vi "LabVIEW_MQTT_Toolkit_V2.vi"() -> ()   [LabVIEW 2021] (continued)
            n1097 = Array Subset(array=w2829, index=2, length=8) -> (w2869:u8[])
            n1098 = Subtract(x=w2830, y=36) -> (x-y=w2825:i32)
            n1099 = Unbundle By Name(w2864) -> ("[0]"=w2863:u8)
            n1100 = Array To Cluster(array=w2869) -> (cluster=w2868:T12)
            n1101 = Unbundle By Name(w2859) -> ("[0]"=w2858:u8, "[1]"=w2729:u8, "[2]"=w2857:u8, "[3]"=w2854:u8, "[4]"=w2853:u8, "[5]"=w2851:u8, "[6]"=w2850:u8, "[7]"=w2849:u8, "[8]"=w2846:u8, "[9]"=w2845:u8, "[10]"=w2844:u8, "[11]"=w2841:u8, "[12]"=w2840:u8, "[13]"=w2834:u8, "[14]"=→"Network quality (LQI)":u8, "[15]"=w2726:u8, "[16]"=w2712:u8, "[17]"=w2711:u8, "[18]"=w2710:u8, "[19]"=w2709:u8, "[20]"=w2702:u8, "[21]"=w2701:u8)
            n1102 = Array Subset(array=w2829, index=36, length=w2825) -> (w2827:u8[])
            n1103 = Unbundle By Name(w2868) -> ("[0]"=w2810:u8, "[1]"=w2811:u8, "[2]"=w2814:u8, "[3]"=w2815:u8, "[4]"=w2808:u8, "[5]"=w2809:u8, "[6]"=w2817:u8, "[7]"=w2816:u8)
            n1104 = case shown="Default" w2726 {
              tunnel: ["channel Z" "channel X" _ "channel Y"] -> w2725
              frame 0 {
              }
              frame 1 {
              }
              frame Default {
              }
              frame 2 {
              }
            }
            "Shock source" <- w2725
            n1105 = Join Numbers "time"(hi=w2811, lo=w2810) -> ((hi.lo)=w2807:u16)
            n1106 = Join Numbers "date"(hi=w2815, lo=w2814) -> ((hi.lo)=w2813:u16)
            n1107 = Join Numbers(hi=w2850, lo=w2851) -> ((hi.lo)=w2848:u16)
            n1108 = Join Numbers(hi=w2845, lo=w2846) -> ((hi.lo)=w2843:u16)
            n1109 = Join Numbers(hi=w2816, lo=w2817) -> ((hi.lo)=w2818:u16)
            n1110 = Join Numbers(hi=w2853, lo=w2854) -> ((hi.lo)=w2852:u16)
            n1111 = Join Numbers(hi=w2729, lo=w2858) -> ((hi.lo)=w2856:u16)
            n1112 = Join Numbers(hi=w2840, lo=w2841) -> ((hi.lo)=w2839:u16)
            n1113 = Join Numbers(hi=w2711, lo=w2712) -> ((hi.lo)=w2720:u16)
            n1114 = Join Numbers(hi=w2709, lo=w2710) -> ((hi.lo)=w2714:u16)
            n1115 = Join Numbers(hi=w2701, lo=w2702) -> ((hi.lo)=w2704:u16)
            n1116 = Join Numbers(hi=w2809, lo=w2808) -> ((hi.lo)=w2800:u16)
            "millisec" <- w2800
            n1117 = Not Equal To 0?(x=w2834) -> (x != 0?=→"synchronised":bool)
            n1118 = Equal To 0?(x=w2834) -> (x = 0?=→"not synchronised":bool)
            n1119 = Decimate 1D Array(w2827) -> (w2820:u8[], w2826:u8[], w2824:u8[])
            n1120 = Join Numbers(hi=w2849, lo=w2848) -> ((hi.lo)=w2847:u32)
            n1121 = Join Numbers(hi=w2844, lo=w2843) -> ((hi.lo)=w2842:u32)
            n1122 = Join Numbers(hi=w2826, lo=w2820) -> ((hi.lo)=w2823:u16[])
            n1123 = Join Numbers(hi=w2857, lo=w2856) -> ((hi.lo)=w2855:u32)
            n1124 = To Word Integer(number=w2839) -> (16bit integer=→"Prev.number of daq per channel":i16)
            n1125 = To Word Integer(number=w2720) -> (16bit integer=w2719:i16)
            n1126 = To Word Integer(number=w2714) -> (16bit integer=w2713:i16)
            n1127 = To Word Integer(number=w2704) -> (16bit integer=w2703:i16)
            n1128 = To Word Integer(number=w2852) -> (16bit integer=w2821:i16)
            "Number of daq per channel" <- w2821
            n1129 = And(x=w2713, y=w2715) -> (x .and. y?=w2716:i16)
            n1130 = And(x=w2703, y=w2705) -> (x .and. y?=w2706:i16)
            n1131 = And(x=w2719, y=w2721) -> (x .and. y?=w2722:i16)
            n1132 = To Long Integer(number=w2847) -> (32bit integer=w2751:i32)
            "Data monitoring cycle" <- w2751
            n1133 = To Long Integer(number=w2842) -> (32bit integer=w2752:i32)
            "Data acquisition duration" <- w2752
            n1134 = To Long Integer(number=w2855) -> (32bit integer=w2822:i32)
            "Frame sequence Id" <- w2822
            n1135 = Divide(x=w2800, y=i16 1000) -> (x/y=w2801:dbl)
            n1136 = for {
              tunnel: w2824 -> [w3352] mode=indexing
              tunnel: [w3350] -> w2780 mode=indexing
              tunnel: w2823 -> [w3348] mode=indexing
              n1137 = To Word Integer(number=w3352) -> (16bit integer=w3349:i16)
              n1138 = Sign(1:w3349) -> (0:w3351:i16)
              n1139 = case shown="1" w3351 {
                tunnel: [_ w3354 w3357] -> w3350
                tunnel: w3348 -> [_ w3353 w3356]
                frame Default {
                }
                frame 1 {
                  n1140 = Divide(x=w3353, y=-1000.0) -> (x/y=w3354:dbl)
                }
                frame 0 {
                  n1141 = Divide(x=w3356, y=1000.0) -> (x/y=w3357:dbl)
                }
              }
            }
            n1142 = And(x=i16 -32768 ("Numeric"), y=w2722) -> (x .and. y?=w2723:i16)
            n1143 = To Unsigned Word Integer(number=w2801) -> (unsigned 16bit integer=w2805:u16)
            n1144 = case shown="4" w2837 {
              tunnel: ["" "LDCDA mode" "Shock Detection"] -> w2775
              tunnel: w2752 -> [_ _ _]
              tunnel: w2751 -> [_ _ _]
              frame Default {
              }
              frame 1 {
              }
              frame 4 {
              }
            }
            n1145 = case shown="0" w2723 {
              tunnel: [w2889 w2890] -> w2699
              tunnel: w2722 -> [w2889 w2895]
              tunnel: w2721 -> [_ w2891]
              frame 0 {
                # "positive"
              }
              frame Default {
                # "negative"
                n1146 = Not(x=w2895) -> (.not. x?=w2894:i16)
                n1147 = And(x=w2894, y=w2891) -> (x .and. y?=w2892:i16)
                n1148 = Increment(x=w2892) -> (x+1=w2893:i16)
                n1149 = Negate(x=w2893) -> (-x=w2890:i16)
              }
            }
            n1150 = Multiply(x=w2821, y=w2822) -> (x*y=w2794:i32)
            n1151 = And(x=i16 -32768 ("Numeric"), y=w2716) -> (x .and. y?=w2717:i16)
            n1152 = And(x=i16 -32768 ("Numeric"), y=w2706) -> (x .and. y?=w2707:i16)
            n1153 = Add(x=w2807, y=w2805) -> (x+y=w2779:u16)
            n1154 = To Unsigned Word Integer(number=w2813) -> (unsigned 16bit integer=w2778:u16)
            n1155 = case shown="0" w2717 {
              tunnel: [w2882 w2883] -> w2695
              tunnel: w2716 -> [w2882 w2888]
              tunnel: w2715 -> [_ w2884]
              frame 0 {
                # "positive"
              }
              frame Default {
                # "negative"
                n1156 = Not(x=w2888) -> (.not. x?=w2887:i16)
                n1157 = And(x=w2887, y=w2884) -> (x .and. y?=w2885:i16)
                n1158 = Increment(x=w2885) -> (x+1=w2886:i16)
                n1159 = Negate(x=w2886) -> (-x=w2883:i16)
              }
            }
            n1160 = case shown="0" w2707 {
              tunnel: [w2875 w2876] -> w2692
              tunnel: w2706 -> [w2875 w2881]
              tunnel: w2705 -> [_ w2877]
              frame 0 {
                # "positive"
              }
              frame Default {
                # "negative"
                n1161 = Not(x=w2881) -> (.not. x?=w2880:i16)
                n1162 = And(x=w2880, y=w2877) -> (x .and. y?=w2878:i16)
                n1163 = Increment(x=w2878) -> (x+1=w2879:i16)
                n1164 = Negate(x=w2879) -> (-x=w2876:i16)
              }
            }
            n1165 = Join Numbers(hi=w2778, lo=w2779) -> ((hi.lo)=w2812:u32)
            n1166 = To Unsigned Byte Integer(number=w2863) -> (unsigned 8bit integer=w2782:u8)
            n1167 = To Unsigned Quad Integer(1:w2794) -> (0:w2793:u64)
            n1168 = case shown="6" w2796 {
              tunnel: ["AX-3D" "HI_INC_MONO" "HI_INC_BI" "X_INC_MONO " "X _INC_BI " "AX_3DS" ""] -> w2727
              frame 1 {
              }
              frame 2 {
              }
              frame 3 {
              }
              frame 4 {
              }
              frame 5 {
              }
              frame 6 {
              }
              frame Default {
              }
            }
            "Device type" <- w2727
            n1169 = To Unsigned Quad Integer(1:w2812) -> (0:w2806:u64)
            n1170 = Increment(x=w2793) -> (x+1=w2797:u64)
            n1171 = for {
              N: w2797 -> [_]
              tunnel: w2793 -> [w3347]
              tunnel: [w3347] -> w2799
            }
            n1172 = call "Unix Time to Timestamp.vi"("Fractional Second"=w2801, "Unix Time (s)"=w2806) -> ("Timestamp"=w2803:timestamp)  [unwired: 8 in, 1 out]
            n1173 = To Word Integer(number=w2818) -> (16bit integer=w2753:i16)
            "Sampling rate" <- w2753
            n1174 = Format Date/Time String(time format string (%c)="%x %X %3u", seconds (now)=w2803, UTC format=TRUE) -> (date/time string=w2745:string)
            "Ref time" <- w2745
            n1175 = Decrement(x=w2799) -> (x-1=w2798:u64)
            n1176 = call <vilib>:"Space Constant.vi"() -> ("String"=w2700:string)
            n1177 = Search and Replace String(replace all?=TRUE ("replace all? (F)"), input string=w2745, search string=":", replace string="_") -> (result string=w2766:string)  [unwired: 4 in, 3 out]
            n1178 = Divide(x=w2699, y=i16 1000) -> (x/y=→"Y Axis first data":dbl)
            n1179 = Number To Decimal String(number=w2753) -> (decimal integer string=w2742:string)  [unwired: 1 in]
            n1180 = Number To Decimal String(number=w2751) -> (decimal integer string=w2739:string)  [unwired: 1 in]
            n1181 = Number To Decimal String(number=w2752) -> (decimal integer string=w2736:string)  [unwired: 1 in]
            n1182 = Concatenate Strings(w2775, w2700) -> (w2728:string)
            "Measure mode" <- w2728
            n1183 = for {
              tunnel: w2780 -> [w3346] mode=indexing
              shift-right: [w3344] -> _
              shift-left: w2798 -> [w3345]
              tunnel: [w3343] -> w2795 mode=indexing
              tunnel: [w3346] -> _ mode=indexing
              n1184 = Increment(x=w3345) -> (x+1=w3344:u64)
              n1185 = To Unsigned Quad Integer(1:w3344) -> (0:w3343:u64)
            }
            n1186 = Search and Replace String(replace all?=TRUE ("replace all? (F)"), input string=w2766, search string=",", replace string="_") -> (result string=w2765:string)  [unwired: 4 in, 3 out]
            n1187 = Divide(x=w2695, y=i16 1000) -> (x/y=→"X Axis first data":dbl)
            n1188 = Divide(x=w2692, y=i16 1000) -> (x/y=→"Z Axis first data":dbl)
            n1189 = Concatenate Strings("Device type :", w2727, ";", "Measure Mode :", w2728, ";", "Reference time :" ("string"), w2745, ";", " Sampling rate :", w2742, ";" ("string"), "Data monitoring cycle" ("string"), w2739, ";" ("string"), "Data acquisition duration :" ("string"), w2736, ";" ("string"), "\n") -> (w2755:string)
            n1190 = Search and Replace String(replace all?=TRUE ("replace all? (F)"), input string=w2765, search string="/", replace string="_") -> (result string=w2761:string)  [unwired: 4 in, 3 out]
            n1191 = String Subset(string=w2761, offset (0)=0, length (rest)=20 ("length (rest)")) -> (substring=w2758:string)
            n1192 = To Double Precision Float(number=w2753) -> (double precision float=w2776:dbl)
            n1193 = Build Array(w2755) -> (w2750:string[])
            n1194 = call <vilib>:"Space Constant.vi"() -> ("String"=w2757:string)
            n1195 = Concatenate Strings(w2758, "_" ("string"), w2730, w2757) -> (w2771:string)
            n1196 = To Unsigned Quad Integer(1:w2795) -> (0:w2777:u64[])
            n1197 = case shown="101" w2782 {
              tunnel: ["" "no active channel" "chZ " "chX  " "chZ & chX " "chY" "chZ & chY  " "chX & chY " "chZ& chX& chY "] -> w2781
              tunnel: w2780 -> [_ _ w2935 w2994 w3055 w3117 w3179 w3244 w3312]
              tunnel: [_ _ w2932 w2991 w3051 w3114 w3177 w3240 w3308] -> w2754
              tunnel: w2777 -> [_ _ w2934 w2993 w3054 w3115 w3178 w3243 w3307]
              tunnel: [_ _ w2931 _ w3050 _ w3174 _ w3306] -> w2788
              tunnel: [_ _ _ w2990 w3049 _ _ w3239 w3305] -> w2787
              tunnel: [_ _ _ _ _ w3113 w3173 w3238 w3304] -> w2786
              tunnel: w2779 -> [_ _ w2930 w2988 w3047 w3111 w3171 w3236 w3302]
              tunnel: w2778 -> [_ _ w2929 w2989 w3048 w3112 w3172 w3237 w3303]
              tunnel: w2777 -> [_ _ w2928 w2987 w3046 w3110 w3170 w3235 w3301]
              tunnel: w2776 -> [_ _ w2927 w2986 w3045 w3109 w3169 w3234 w3300]
              tunnel: [_ _ w2926 _ w3044 _ w3168 _ w3299] -> w2785
              tunnel: [_ _ _ w2985 w3044 _ _ w3233 w3298] -> w2784
              tunnel: [_ _ _ _ _ w3108 w3167 w3232 w3297] -> w2783
              tunnel: w2771 -> [_ _ w2912 w2962 w3021 w3085 w3143 w3209 w3274]
              tunnel: [_ _ w2902 w2961 w3020 w3084 w3144 w3208 w3273] -> w2689
              tunnel: w2750 -> [_ _ w2901 w2960 w3019 w3083 w3142 w3207 w3272]
              frame Default {
              }
              frame 0 {
              }
              frame 1 {
                w2907 = T14 2 items=["User Home"=0, "User Desktop"=1, "User Documents"=2, "User Application Data"=3, "User Preferences"=4, "User Temporary"=5, "Public Documents"=6, "Public Application Data"=7, "Public Preferences"=8, "Public Cache"=13, "System Core Libraries"=9, "System Installed Libraries"=10, "Application Files"=11, "Boot Volume Root"=12] ("system directory type")
                n1198 = Decimate 1D Array(w2935) -> (w2933:dbl[])
                n1199 = Search and Replace String(replace all?=TRUE ("replace all? (F)"), input string=w2912, search string="/") -> (result string=w2924:string)  [unwired: 5 in, 3 out]
                n1200 = Concatenate Strings(w2901, "TimeStamp;MeasureCh_Z(g);", "\n") -> (w2917:string)
                n1201 = for {
                  tunnel: w2933 -> [w2954] mode=indexing
                  tunnel: [w2957] -> w2932 mode=indexing
                  tunnel: w2934 -> [w2956] mode=indexing
                  tunnel: [w2954] -> w2931 mode=indexing
                  tunnel: w2930 -> [w2949]
                  tunnel: w2929 -> [w2948]
                  tunnel: w2928 -> [w2947] mode=indexing
                  tunnel: w2927 -> [w2946]
                  tunnel: [w2940] -> w2926
                  n1202 = Join Numbers(hi=w2948, lo=w2949) -> ((hi.lo)=w2951:u32)
                  n1203 = To Double Precision Float(number=w2947) -> (double precision float=w2952:dbl)
                  n1204 = Number To Decimal String(number=w2956) -> (decimal integer string=w2955:string)  [unwired: 1 in]
                  n1205 = Number To Fractional String(number=w2954, precision (6)=i16 3 ("width (-)")) -> (F-format string=w2958:string)  [unwired: 2 in]
                  n1206 = Divide(x=w2952, y=w2946) -> (x/y=w2953:dbl)
                  n1207 = Build Array(w2955, w2958) -> (w2957:string[])
                  n1208 = To Unsigned Quad Integer(1:w2951) -> (0:w2950:u64)
                  n1209 = call "Unix Time to Timestamp.vi"("Fractional Second"=w2953, "Unix Time (s)"=w2950) -> ("Timestamp"=w2941:timestamp)  [unwired: 8 in, 1 out]
                  n1210 = Format Date/Time String(seconds (now)=w2941, UTC format=TRUE) -> (date/time string=w2942:string)  [unwired: 1 in]
                  n1211 = Scan From String(format string="%<%x %H:%M:%S%3u>T", input string=w2942) -> (output 1=w2943:timestamp)  [unwired: 3 in, 3 out]
                  n1212 = To Double Precision Float(number=w2943) -> (double precision float=w2940:dbl)
                }
                n1213 = call <vilib>:"Get System Directory.vi"("system directory type"=w2907) -> ("system directory"=w2918:path)  [unwired: 10 in]
                n1214 = Concatenate Strings(w2924, "_" ("string"), "ShockDetection.csv") -> (w2925:string)
                n1215 = Build Path(base path=w2918, name or relative path="Logfile") -> (appended path=w2919:path)
                n1216 = call <vilib>:"Check if File or Folder Exists.vi"("path"=w2919) -> ("file or folder exists?"=w2920:bool, "dup path"=w2921:path)  [unwired: 8 in, 1 out]
                n1217 = case shown="False" w2920 {
                  tunnel: w2921 -> [w2938 w2939]
                  tunnel: [w2937 w2939] -> w2922
                  frame False {
                    n1218 = Create Folder(path (use dialog)=w2938) -> (created path=w2937:path)  [unwired: 2 in, 2 out]
                  }
                  frame True {
                  }
                }
                n1219 = Build Path(base path=w2922, name or relative path=w2925) -> (appended path=w2923:path)
                n1220 = Open/Create/Replace File(file path (use dialog)=w2923, operation (0:open)=T11."open or create") -> (refnum out=w2916:refnum<file>, error out=w2914:errorcluster)  [unwired: 4 in, 1 out]
                n1221 = Write to Text File(file (use dialog)=w2916, text=w2917, error in=w2914) -> (refnum out=w2915:refnum<file>, error out=w2913:errorcluster)  [unwired: 1 in, 1 out]
                n1222 = Close File(refnum=w2915, error in=w2913) -> (path=w2902:path)  [unwired: 1 out]
              }
              frame 2 {
                w2967 = T14 2 items=["User Home"=0, "User Desktop"=1, "User Documents"=2, "User Application Data"=3, "User Preferences"=4, "User Temporary"=5, "Public Documents"=6, "Public Application Data"=7, "Public Preferences"=8, "Public Cache"=13, "System Core Libraries"=9, "System Installed Libraries"=10, "Application Files"=11, "Boot Volume Root"=12] ("system directory type")
                n1223 = Decimate 1D Array(w2994) -> (w2992:dbl[])
                n1224 = Search and Replace String(replace all?=TRUE ("replace all? (F)"), input string=w2962, search string="/") -> (result string=w2983:string)  [unwired: 5 in, 3 out]
                n1225 = for {
                  tunnel: w2992 -> [w3013] mode=indexing
                  tunnel: [w3016] -> w2991 mode=indexing
                  tunnel: w2993 -> [w3015] mode=indexing
                  tunnel: [w3013] -> w2990 mode=indexing
                  tunnel: w2989 -> [w3008]
                  tunnel: w2988 -> [w3007]
                  tunnel: w2987 -> [w3006] mode=indexing
                  tunnel: w2986 -> [w3005]
                  tunnel: [w2999] -> w2985
                  n1226 = Join Numbers(hi=w3008, lo=w3007) -> ((hi.lo)=w3010:u32)
                  n1227 = To Double Precision Float(number=w3006) -> (double precision float=w3011:dbl)
                  n1228 = Number To Decimal String(number=w3015) -> (decimal integer string=w3014:string)  [unwired: 1 in]
                  n1229 = Number To Fractional String(number=w3013, precision (6)=i16 3 ("width (-)")) -> (F-format string=w3017:string)  [unwired: 2 in]
                  n1230 = Divide(x=w3011, y=w3005) -> (x/y=w3012:dbl)
                  n1231 = Build Array(w3014, w3017) -> (w3016:string[])
                  n1232 = To Unsigned Quad Integer(1:w3010) -> (0:w3009:u64)
                  n1233 = call "Unix Time to Timestamp.vi"("Fractional Second"=w3012, "Unix Time (s)"=w3009) -> ("Timestamp"=w3000:timestamp)  [unwired: 8 in, 1 out]
                  n1234 = Format Date/Time String(seconds (now)=w3000, UTC format=TRUE) -> (date/time string=w3001:string)  [unwired: 1 in]
                  n1235 = Scan From String(format string="%<%x %H:%M:%S%3u>T", input string=w3001) -> (output 1=w3002:timestamp)  [unwired: 3 in, 3 out]
                  n1236 = To Double Precision Float(number=w3002) -> (double precision float=w2999:dbl)
                }
                n1237 = Concatenate Strings(w2960, "TimeStamp;MeasureCh_X(g);", "\n") -> (w2976:string)
                n1238 = call <vilib>:"Get System Directory.vi"("system directory type"=w2967) -> ("system directory"=w2977:path)  [unwired: 10 in]
                n1239 = Concatenate Strings(w2983, "_" ("string"), "ShockDetection.csv") -> (w2984:string)
                n1240 = Build Path(base path=w2977, name or relative path="Logfile") -> (appended path=w2978:path)
                n1241 = call <vilib>:"Check if File or Folder Exists.vi"("path"=w2978) -> ("file or folder exists?"=w2979:bool, "dup path"=w2980:path)  [unwired: 8 in, 1 out]
                n1242 = case shown="False" w2979 {
                  tunnel: w2980 -> [w2997 w2998]
                  tunnel: [w2996 w2998] -> w2981
                  frame False {
                    n1243 = Create Folder(path (use dialog)=w2997) -> (created path=w2996:path)  [unwired: 2 in, 2 out]
                  }
                  frame True {
                  }
                }
                n1244 = Build Path(base path=w2981, name or relative path=w2984) -> (appended path=w2982:path)
                n1245 = Open/Create/Replace File(file path (use dialog)=w2982, operation (0:open)=T11."open or create") -> (refnum out=w2975:refnum<file>, error out=w2973:errorcluster)  [unwired: 4 in, 1 out]
                n1246 = Write to Text File(file (use dialog)=w2975, text=w2976, error in=w2973) -> (refnum out=w2974:refnum<file>, error out=w2972:errorcluster)  [unwired: 1 in, 1 out]
                n1247 = Close File(refnum=w2974, error in=w2972) -> (path=w2961:path)  [unwired: 1 out]
              }
              frame 3 {
                w3026 = T14 2 items=["User Home"=0, "User Desktop"=1, "User Documents"=2, "User Application Data"=3, "User Preferences"=4, "User Temporary"=5, "Public Documents"=6, "Public Application Data"=7, "Public Preferences"=8, "Public Cache"=13, "System Core Libraries"=9, "System Installed Libraries"=10, "Application Files"=11, "Boot Volume Root"=12] ("system directory type")
                n1248 = Decimate 1D Array(w3055) -> (w3053:dbl[], w3052:dbl[])
                n1249 = Search and Replace String(replace all?=TRUE ("replace all? (F)"), input string=w3021, search string="/") -> (result string=w3042:string)  [unwired: 5 in, 3 out]
                n1250 = for {
                  tunnel: w3053 -> [w3075] mode=indexing
                  tunnel: w3052 -> [w3074] mode=indexing
                  tunnel: [w3078] -> w3051 mode=indexing
                  tunnel: w3054 -> [w3077] mode=indexing
                  tunnel: [w3075] -> w3050 mode=indexing
                  tunnel: [w3074] -> w3049 mode=indexing
                  tunnel: w3048 -> [w3069]
                  tunnel: w3047 -> [w3068]
                  tunnel: w3046 -> [w3067] mode=indexing
                  tunnel: w3045 -> [w3066]
                  tunnel: [w3060] -> w3044
                  n1251 = Join Numbers(hi=w3069, lo=w3068) -> ((hi.lo)=w3071:u32)
                  n1252 = To Double Precision Float(number=w3067) -> (double precision float=w3072:dbl)
                  n1253 = Number To Decimal String(number=w3077) -> (decimal integer string=w3076:string)  [unwired: 1 in]
                  n1254 = Number To Fractional String(number=w3075, precision (6)=i16 3 ("width (-)")) -> (F-format string=w3080:string)  [unwired: 2 in]
                  n1255 = Number To Fractional String(number=w3074, precision (6)=i16 3 ("width (-)")) -> (F-format string=w3079:string)  [unwired: 2 in]
                  n1256 = Divide(x=w3072, y=w3066) -> (x/y=w3073:dbl)
                  n1257 = Build Array(w3076, w3080, w3079) -> (w3078:string[])
                  n1258 = To Unsigned Quad Integer(1:w3071) -> (0:w3070:u64)
                  n1259 = call "Unix Time to Timestamp.vi"("Fractional Second"=w3073, "Unix Time (s)"=w3070) -> ("Timestamp"=w3061:timestamp)  [unwired: 8 in, 1 out]
                  n1260 = Format Date/Time String(seconds (now)=w3061, UTC format=TRUE) -> (date/time string=w3062:string)  [unwired: 1 in]
                  n1261 = Scan From String(format string="%<%x %H:%M:%S%3u>T", input string=w3062) -> (output 1=w3063:timestamp)  [unwired: 3 in, 3 out]
                  n1262 = To Double Precision Float(number=w3063) -> (double precision float=w3060:dbl)
                }
                n1263 = Concatenate Strings(w3019, "TimeStamp;MeasureCh_Z(g);Ch_X(g);", "\n") -> (w3035:string)
                n1264 = call <vilib>:"Get System Directory.vi"("system directory type"=w3026) -> ("system directory"=w3036:path)  [unwired: 10 in]
                n1265 = Concatenate Strings(w3042, "_" ("string"), "ShockDetection.csv") -> (w3043:string)
                n1266 = Build Path(base path=w3036, name or relative path="Logfile") -> (appended path=w3037:path)
                n1267 = call <vilib>:"Check if File or Folder Exists.vi"("path"=w3037) -> ("file or folder exists?"=w3038:bool, "dup path"=w3039:path)  [unwired: 8 in, 1 out]
                n1268 = case shown="False" w3038 {
                  tunnel: w3039 -> [w3058 w3059]
                  tunnel: [w3057 w3059] -> w3040
                  frame False {
                    n1269 = Create Folder(path (use dialog)=w3058) -> (created path=w3057:path)  [unwired: 2 in, 2 out]
                  }
                  frame True {
                  }
                }
                n1270 = Build Path(base path=w3040, name or relative path=w3043) -> (appended path=w3041:path)
                n1271 = Open/Create/Replace File(file path (use dialog)=w3041, operation (0:open)=T11."open or create") -> (refnum out=w3034:refnum<file>, error out=w3032:errorcluster)  [unwired: 4 in, 1 out]
                n1272 = Write to Text File(file (use dialog)=w3034, text=w3035, error in=w3032) -> (refnum out=w3033:refnum<file>, error out=w3031:errorcluster)  [unwired: 1 in, 1 out]
                n1273 = Close File(refnum=w3033, error in=w3031) -> (path=w3020:path)  [unwired: 1 out]
              }
              frame 4 {
                w3090 = T14 2 items=["User Home"=0, "User Desktop"=1, "User Documents"=2, "User Application Data"=3, "User Preferences"=4, "User Temporary"=5, "Public Documents"=6, "Public Application Data"=7, "Public Preferences"=8, "Public Cache"=13, "System Core Libraries"=9, "System Installed Libraries"=10, "Application Files"=11, "Boot Volume Root"=12] ("system directory type")
                n1274 = Decimate 1D Array(w3117) -> (w3116:dbl[])
                n1275 = Search and Replace String(replace all?=TRUE ("replace all? (F)"), input string=w3085, search string="/") -> (result string=w3106:string)  [unwired: 5 in, 3 out]
                n1276 = for {
                  tunnel: w3116 -> [w3136] mode=indexing
                  tunnel: [w3139] -> w3114 mode=indexing
                  tunnel: w3115 -> [w3138] mode=indexing
                  tunnel: [w3136] -> w3113 mode=indexing
                  tunnel: w3112 -> [w3131]
                  tunnel: w3111 -> [w3128]
                  tunnel: w3110 -> [w3129] mode=indexing
                  tunnel: w3109 -> [w3130]
                  tunnel: [w3122] -> w3108
                  n1277 = Join Numbers(hi=w3131, lo=w3128) -> ((hi.lo)=w3133:u32)
                  n1278 = To Double Precision Float(number=w3129) -> (double precision float=w3134:dbl)
                  n1279 = Number To Decimal String(number=w3138) -> (decimal integer string=w3137:string)  [unwired: 1 in]
                  n1280 = Number To Fractional String(number=w3136, precision (6)=i16 3 ("width (-)")) -> (F-format string=w3140:string)  [unwired: 2 in]
                  n1281 = Divide(x=w3134, y=w3130) -> (x/y=w3135:dbl)
                  n1282 = Build Array(w3137, w3140) -> (w3139:string[])
                  n1283 = To Unsigned Quad Integer(1:w3133) -> (0:w3132:u64)
                  n1284 = call "Unix Time to Timestamp.vi"("Fractional Second"=w3135, "Unix Time (s)"=w3132) -> ("Timestamp"=w3123:timestamp)  [unwired: 8 in, 1 out]
                  n1285 = Format Date/Time String(seconds (now)=w3123, UTC format=TRUE) -> (date/time string=w3124:string)  [unwired: 1 in]
                  n1286 = Scan From String(format string="%<%x %H:%M:%S%3u>T", input string=w3124) -> (output 1=w3125:timestamp)  [unwired: 3 in, 3 out]
                  n1287 = To Double Precision Float(number=w3125) -> (double precision float=w3122:dbl)
                }
                n1288 = Concatenate Strings(w3083, "TimeStamp;MeasureCh_Y(g);", "\n") -> (w3099:string)
                n1289 = call <vilib>:"Get System Directory.vi"("system directory type"=w3090) -> ("system directory"=w3100:path)  [unwired: 10 in]
                n1290 = Concatenate Strings(w3106, "_" ("string"), "ShockDetection.csv") -> (w3107:string)
                n1291 = Build Path(base path=w3100, name or relative path="Logfile") -> (appended path=w3101:path)
                n1292 = call <vilib>:"Check if File or Folder Exists.vi"("path"=w3101) -> ("file or folder exists?"=w3102:bool, "dup path"=w3103:path)  [unwired: 8 in, 1 out]
                n1293 = case shown="False" w3102 {
                  tunnel: w3103 -> [w3120 w3121]
                  tunnel: [w3119 w3121] -> w3104
                  frame False {
                    n1294 = Create Folder(path (use dialog)=w3120) -> (created path=w3119:path)  [unwired: 2 in, 2 out]
                  }
                  frame True {
                  }
                }
                n1295 = Build Path(base path=w3104, name or relative path=w3107) -> (appended path=w3105:path)
                n1296 = Open/Create/Replace File(file path (use dialog)=w3105, operation (0:open)=T11."open or create") -> (refnum out=w3098:refnum<file>, error out=w3096:errorcluster)  [unwired: 4 in, 1 out]
                n1297 = Write to Text File(file (use dialog)=w3098, text=w3099, error in=w3096) -> (refnum out=w3097:refnum<file>, error out=w3095:errorcluster)  [unwired: 1 in, 1 out]
                n1298 = Close File(refnum=w3097, error in=w3095) -> (path=w3084:path)  [unwired: 1 out]
              }
              frame 5 {
                w3149 = T14 2 items=["User Home"=0, "User Desktop"=1, "User Documents"=2, "User Application Data"=3, "User Preferences"=4, "User Temporary"=5, "Public Documents"=6, "Public Application Data"=7, "Public Preferences"=8, "Public Cache"=13, "System Core Libraries"=9, "System Installed Libraries"=10, "Application Files"=11, "Boot Volume Root"=12] ("system directory type")
                n1299 = Decimate 1D Array(w3179) -> (w3175:dbl[], w3176:dbl[])
                n1300 = Search and Replace String(replace all?=TRUE ("replace all? (F)"), input string=w3143, search string="/") -> (result string=w3165:string)  [unwired: 5 in, 3 out]
                n1301 = Concatenate Strings(w3142, "TimeStamp;MeasureCh_Z(g);Ch_Y(g);", "\n") -> (w3158:string)
                n1302 = for {
                  tunnel: [w3202] -> w3177 mode=indexing
                  tunnel: w3178 -> [w3201] mode=indexing
                  tunnel: w3175 -> [w3199] mode=indexing
                  tunnel: w3176 -> [w3198] mode=indexing
                  tunnel: [w3199] -> w3174 mode=indexing
                  tunnel: [w3198] -> w3173 mode=indexing
                  tunnel: w3172 -> [w3193]
                  tunnel: w3171 -> [w3192]
                  tunnel: w3170 -> [w3191] mode=indexing
                  tunnel: w3169 -> [w3190]
                  tunnel: [w3184] -> w3168
                  tunnel: [w3184] -> w3167
                  n1303 = Join Numbers(hi=w3193, lo=w3192) -> ((hi.lo)=w3195:u32)
                  n1304 = To Double Precision Float(number=w3191) -> (double precision float=w3196:dbl)
                  n1305 = Number To Decimal String(number=w3201) -> (decimal integer string=w3200:string)  [unwired: 1 in]
                  n1306 = Number To Fractional String(number=w3199, precision (6)=i16 3 ("width (-)")) -> (F-format string=w3204:string)  [unwired: 2 in]
                  n1307 = Number To Fractional String(number=w3198, precision (6)=i16 3 ("width (-)")) -> (F-format string=w3203:string)  [unwired: 2 in]
                  n1308 = Divide(x=w3196, y=w3190) -> (x/y=w3197:dbl)
                  n1309 = Build Array(w3200, w3204, w3203) -> (w3202:string[])
                  n1310 = To Unsigned Quad Integer(1:w3195) -> (0:w3194:u64)
                  n1311 = call "Unix Time to Timestamp.vi"("Fractional Second"=w3197, "Unix Time (s)"=w3194) -> ("Timestamp"=w3185:timestamp)  [unwired: 8 in, 1 out]
                  n1312 = Format Date/Time String(seconds (now)=w3185, UTC format=TRUE) -> (date/time string=w3189:string)  [unwired: 1 in]
                  n1313 = Scan From String(format string="%<%x %H:%M:%S%3u>T", input string=w3189) -> (output 1=w3188:timestamp)  [unwired: 3 in, 3 out]
                  n1314 = To Double Precision Float(number=w3188) -> (double precision float=w3184:dbl)
                }
                n1315 = call <vilib>:"Get System Directory.vi"("system directory type"=w3149) -> ("system directory"=w3159:path)  [unwired: 10 in]
                n1316 = Concatenate Strings(w3165, "_" ("string"), "ShockDetection.csv") -> (w3166:string)
                n1317 = Build Path(base path=w3159, name or relative path="Logfile") -> (appended path=w3160:path)
                n1318 = call <vilib>:"Check if File or Folder Exists.vi"("path"=w3160) -> ("file or folder exists?"=w3161:bool, "dup path"=w3162:path)  [unwired: 8 in, 1 out]
                n1319 = case shown="False" w3161 {
                  tunnel: w3162 -> [w3182 w3183]
                  tunnel: [w3181 w3183] -> w3163
                  frame False {
                    n1320 = Create Folder(path (use dialog)=w3182) -> (created path=w3181:path)  [unwired: 2 in, 2 out]
                  }
                  frame True {
                  }
                }
                n1321 = Build Path(base path=w3163, name or relative path=w3166) -> (appended path=w3164:path)
                n1322 = Open/Create/Replace File(file path (use dialog)=w3164, operation (0:open)=T11."open or create") -> (refnum out=w3157:refnum<file>, error out=w3155:errorcluster)  [unwired: 4 in, 1 out]
                n1323 = Write to Text File(file (use dialog)=w3157, text=w3158, error in=w3155) -> (refnum out=w3156:refnum<file>, error out=w3154:errorcluster)  [unwired: 1 in, 1 out]
                n1324 = Close File(refnum=w3156, error in=w3154) -> (path=w3144:path)  [unwired: 1 out]
              }
              frame 6 {
                w3214 = T14 2 items=["User Home"=0, "User Desktop"=1, "User Documents"=2, "User Application Data"=3, "User Preferences"=4, "User Temporary"=5, "Public Documents"=6, "Public Application Data"=7, "Public Preferences"=8, "Public Cache"=13, "System Core Libraries"=9, "System Installed Libraries"=10, "Application Files"=11, "Boot Volume Root"=12] ("system directory type")
                n1325 = Decimate 1D Array(w3244) -> (w3242:dbl[], w3241:dbl[])
                n1326 = Search and Replace String(replace all?=TRUE ("replace all? (F)"), input string=w3209, search string="/") -> (result string=w3230:string)  [unwired: 5 in, 3 out]
                n1327 = for {
                  tunnel: w3242 -> [w3264] mode=indexing
                  tunnel: w3241 -> [w3263] mode=indexing
                  tunnel: [w3267] -> w3240 mode=indexing
                  tunnel: w3243 -> [w3266] mode=indexing
                  tunnel: [w3264] -> w3239 mode=indexing
                  tunnel: [w3263] -> w3238 mode=indexing
                  tunnel: w3237 -> [w3258]
                  tunnel: w3236 -> [w3257]
                  tunnel: w3235 -> [w3256] mode=indexing
                  tunnel: w3234 -> [w3255]
                  tunnel: [w3249] -> w3233
                  tunnel: [w3249] -> w3232
                  n1328 = Join Numbers(hi=w3258, lo=w3257) -> ((hi.lo)=w3260:u32)
                  n1329 = To Double Precision Float(number=w3256) -> (double precision float=w3261:dbl)
                  n1330 = Number To Decimal String(number=w3266) -> (decimal integer string=w3265:string)  [unwired: 1 in]
                  n1331 = Number To Fractional String(number=w3264, precision (6)=i16 3 ("width (-)")) -> (F-format string=w3269:string)  [unwired: 2 in]
                  n1332 = Number To Fractional String(number=w3263, precision (6)=i16 3 ("width (-)")) -> (F-format string=w3268:string)  [unwired: 2 in]
                  n1333 = Divide(x=w3261, y=w3255) -> (x/y=w3262:dbl)
                  n1334 = Build Array(w3265, w3269, w3268) -> (w3267:string[])
                  n1335 = To Unsigned Quad Integer(1:w3260) -> (0:w3259:u64)
                  n1336 = call "Unix Time to Timestamp.vi"("Fractional Second"=w3262, "Unix Time (s)"=w3259) -> ("Timestamp"=w3250:timestamp)  [unwired: 8 in, 1 out]
                  n1337 = Format Date/Time String(seconds (now)=w3250, UTC format=TRUE) -> (date/time string=w3251:string)  [unwired: 1 in]
                  n1338 = Scan From String(format string="%<%x %H:%M:%S%3u>T", input string=w3251) -> (output 1=w3252:timestamp)  [unwired: 3 in, 3 out]
                  n1339 = To Double Precision Float(number=w3252) -> (double precision float=w3249:dbl)
                }
                n1340 = Concatenate Strings(w3207, "TimeStamp;MeasureCh_X(g);Ch_Y(g);", "\n") -> (w3223:string)
                n1341 = call <vilib>:"Get System Directory.vi"("system directory type"=w3214) -> ("system directory"=w3224:path)  [unwired: 10 in]
                n1342 = Concatenate Strings(w3230, "_" ("string"), "ShockDetection.csv") -> (w3231:string)
                n1343 = Build Path(base path=w3224, name or relative path="Logfile") -> (appended path=w3225:path)
                n1344 = call <vilib>:"Check if File or Folder Exists.vi"("path"=w3225) -> ("file or folder exists?"=w3226:bool, "dup path"=w3227:path)  [unwired: 8 in, 1 out]
                n1345 = case shown="False" w3226 {
                  tunnel: w3227 -> [w3247 w3248]
                  tunnel: [w3246 w3248] -> w3228
                  frame False {
                    n1346 = Create Folder(path (use dialog)=w3247) -> (created path=w3246:path)  [unwired: 2 in, 2 out]
                  }
                  frame True {
                  }
                }
                n1347 = Build Path(base path=w3228, name or relative path=w3231) -> (appended path=w3229:path)
                n1348 = Open/Create/Replace File(file path (use dialog)=w3229, operation (0:open)=T11."open or create") -> (refnum out=w3222:refnum<file>, error out=w3220:errorcluster)  [unwired: 4 in, 1 out]
                n1349 = Write to Text File(file (use dialog)=w3222, text=w3223, error in=w3220) -> (refnum out=w3221:refnum<file>, error out=w3219:errorcluster)  [unwired: 1 in, 1 out]
                n1350 = Close File(refnum=w3221, error in=w3219) -> (path=w3208:path)  [unwired: 1 out]
              }
              frame 7 {
                w3279 = T14 2 items=["User Home"=0, "User Desktop"=1, "User Documents"=2, "User Application Data"=3, "User Preferences"=4, "User Temporary"=5, "Public Documents"=6, "Public Application Data"=7, "Public Preferences"=8, "Public Cache"=13, "System Core Libraries"=9, "System Installed Libraries"=10, "Application Files"=11, "Boot Volume Root"=12] ("system directory type")
                n1351 = Search and Replace String(replace all?=TRUE ("replace all? (F)"), input string=w3274, search string="/") -> (result string=w3295:string)  [unwired: 5 in, 3 out]
                n1352 = Concatenate Strings(w3272, "TimeStamp;MeasureCh_Z(g);Ch_X(g);Ch_Y(g);", "\n") -> (w3288:string)
                n1353 = call <vilib>:"Get System Directory.vi"("system directory type"=w3279) -> ("system directory"=w3289:path)  [unwired: 10 in]
                n1354 = Concatenate Strings(w3295, "_" ("string"), "ShockDetection.csv") -> (w3296:string)
                n1355 = Decimate 1D Array(w3312) -> (w3311:dbl[], w3310:dbl[], w3309:dbl[])
                n1356 = for {
                  tunnel: w3311 -> [w3333] mode=indexing
                  tunnel: w3310 -> [w3332] mode=indexing
                  tunnel: w3309 -> [w3331] mode=indexing
                  tunnel: [w3336] -> w3308 mode=indexing
                  tunnel: w3307 -> [w3335] mode=indexing
                  tunnel: [w3333] -> w3306 mode=indexing
                  tunnel: [w3332] -> w3305 mode=indexing
                  tunnel: [w3331] -> w3304 mode=indexing
                  tunnel: w3303 -> [w3326]
                  tunnel: w3302 -> [w3325]
                  tunnel: w3301 -> [w3324] mode=indexing
                  tunnel: w3300 -> [w3323]
                  tunnel: [w3317] -> w3299
                  tunnel: [w3317] -> w3298
                  tunnel: [w3317] -> w3297
                  n1357 = Join Numbers(hi=w3326, lo=w3325) -> ((hi.lo)=w3328:u32)
                  n1358 = To Double Precision Float(number=w3324) -> (double precision float=w3329:dbl)
                  n1359 = Number To Decimal String(number=w3335) -> (decimal integer string=w3334:string)  [unwired: 1 in]
                  n1360 = Number To Fractional String(number=w3333, precision (6)=i16 3 ("width (-)")) -> (F-format string=w3340:string)  [unwired: 2 in]
                  n1361 = Number To Fractional String(number=w3332, precision (6)=i16 3 ("width (-)")) -> (F-format string=w3339:string)  [unwired: 2 in]
                  n1362 = Number To Fractional String(number=w3331, precision (6)=i16 3 ("width (-)")) -> (F-format string=w3337:string)  [unwired: 2 in]
                  n1363 = Build Array(w3334, w3340, w3339, w3337) -> (w3336:string[])
                  n1364 = Divide(x=w3329, y=w3323) -> (x/y=w3330:dbl)
                  n1365 = To Unsigned Quad Integer(1:w3328) -> (0:w3327:u64)
                  n1366 = call "Unix Time to Timestamp.vi"("Fractional Second"=w3330, "Unix Time (s)"=w3327) -> ("Timestamp"=w3318:timestamp)  [unwired: 8 in, 1 out]
                  n1367 = Format Date/Time String(seconds (now)=w3318, UTC format=TRUE) -> (date/time string=w3319:string)  [unwired: 1 in]
                  n1368 = Scan From String(format string="%<%x %H:%M:%S%3u>T", input string=w3319) -> (output 1=w3320:timestamp)  [unwired: 3 in, 3 out]
                  n1369 = To Double Precision Float(number=w3320) -> (double precision float=w3317:dbl)
                }
                n1370 = Build Path(base path=w3289, name or relative path="Logfile") -> (appended path=w3290:path)
                n1371 = call <vilib>:"Check if File or Folder Exists.vi"("path"=w3290) -> ("file or folder exists?"=w3291:bool, "dup path"=w3292:path)  [unwired: 8 in, 1 out]
                n1372 = case shown="False" w3291 {
                  tunnel: w3292 -> [w3315 w3316]
                  tunnel: [w3314 w3316] -> w3293
                  frame False {
                    n1373 = Create Folder(path (use dialog)=w3315) -> (created path=w3314:path)  [unwired: 2 in, 2 out]
                  }
                  frame True {
                  }
                }
                n1374 = Build Path(base path=w3293, name or relative path=w3296) -> (appended path=w3294:path)
                n1375 = Open/Create/Replace File(file path (use dialog)=w3294, operation (0:open)=T11."open or create") -> (refnum out=w3287:refnum<file>, error out=w3285:errorcluster)  [unwired: 4 in, 1 out]
                n1376 = Write to Text File(file (use dialog)=w3287, text=w3288, error in=w3285) -> (refnum out=w3286:refnum<file>, error out=w3284:errorcluster)  [unwired: 1 in, 1 out]
                n1377 = Close File(refnum=w3286, error in=w3284) -> (path=w3273:path)  [unwired: 1 out]
              }
            }
            "Enabled channels" <- w2781
            "CH_Z Graph" <- w2788
            "CH_X Graph" <- w2787
            "CH_Y Graph" <- w2786
            "File path" <- w2689
            n1378 = property on="CH_X Graph" class="WFChart (strict)"("XScale.Offset"=w2784) -> ()  [unwired: 2 in, 2 out]
            n1379 = property on="CH_Z Graph" class="WFChart (strict)"("XScale.Offset"=w2785) -> ()  [unwired: 2 in, 2 out]
            n1380 = property on="CH_Y Graph" class="WFChart (strict)"("XScale.Offset"=w2783) -> ()  [unwired: 2 in, 2 out]
            n1381 = call-poly <vilib>:"Write Delimited Spreadsheet.vi"("file path (dialog if empty)"=w2689, "format (%s)"="%s", "2D data"=w2754, "append to file? (new file:F)"=TRUE, "transpose? (no:F)"=FALSE, "delimiter (\\t)"=";" ("delimiter (\\t)")) -> ()  [unwired: 8 in, 2 out]
          }
          frame 5 {
            w3393 = T14 2 items=["User Home"=0, "User Desktop"=1, "User Documents"=2, "User Application Data"=3, "User Preferences"=4, "User Temporary"=5, "Public Documents"=6, "Public Application Data"=7, "Public Preferences"=8, "Public Cache"=13, "System Core Libraries"=9, "System Installed Libraries"=10, "Application Files"=11, "Boot Volume Root"=12] ("system directory type")
            # "this block contain event date date"
            # "function to write data in log file"
            # "logfile path"
            # "precision"
            # "this block contain start date"
            # "measured value"
            # "this function contain end date"
            # "this block contain mathmode type +date"
            n1382 = case shown="1" w3414 {
              tunnel: [_ w3425 w3428] -> w3397
              tunnel: w3416 -> [_ w3424 w3427]
              frame Default {
              }
              frame 1 {
                n1383 = Divide(x=w3424, y=-1000.0) -> (x/y=w3425:dbl)
              }
              frame 0 {
                n1384 = Divide(x=w3427, y=1000.0) -> (x/y=w3428:dbl)
              }
            }
            n1385 = call "Unix Time to Timestamp.vi"("Unix Time (s)"=w3373) -> ("Timestamp"=w3374:timestamp)  [unwired: 9 in, 1 out]
            n1386 = Format Date/Time String(seconds (now)=w3374, UTC format=TRUE) -> (date/time string=w3376:string)  [unwired: 1 in]
            n1387 = call <vilib>:"Get System Directory.vi"("system directory type"=w3393) -> ("system directory"=w3394:path)  [unwired: 10 in]
            n1388 = Less?(x=w3373, y=w3372) -> (x < y?=w3410:bool)
            n1389 = Select(t="NA                 ", s=w3410, f=w3376) -> (s? t:f=w3395:string)
            n1390 = case shown="1" w3415 {
              tunnel: w3397 -> [w3431 w3434 w3437 _]
              tunnel: w3395 -> [w3432 w3435 _ _]
              tunnel: [w3431 _ _ _] -> _
              tunnel: [_ w3434 _ _] -> _
              tunnel: [_ _ w3437 _] -> _
              tunnel: ["Maximum value" "Minimum value" "Average value" _] -> w3398
              frame 1 {
                "Maximum value" <- w3431
                "Date" <- w3432
              }
              frame 2 {
                "Minimum value" <- w3434
                "Date" <- w3435
              }
              frame 3 {
                "Average value" <- w3437
              }
              frame Default {
              }
            }
            n1391 = Build Path(base path=w3394, name or relative path="Logfile") -> (appended path=w3391:path)
            n1392 = call <vilib>:"Check if File or Folder Exists.vi"("path"=w3391) -> ("file or folder exists?"=w3390:bool, "dup path"=w3389:path)  [unwired: 8 in, 1 out]
            n1393 = call "Unix Time to Timestamp.vi"("Unix Time (s)"=w3417) -> ("Timestamp"=w3412:timestamp)  [unwired: 9 in, 1 out]
            n1394 = call "Unix Time to Timestamp.vi"("Unix Time (s)"=w3372) -> ("Timestamp"=w3411:timestamp)  [unwired: 9 in, 1 out]
            n1395 = String Subset(string=w3378, offset (0)=0, length (rest)=16 ("length (rest)")) -> (substring=w3377:string)
            n1396 = Concatenate Strings(w3377, "_" ("string"), w3383, "_" ("string"), "Transmit_Math_LowDutyCycle.txt") -> (w3386:string)
            n1397 = case shown="False" w3390 {
              tunnel: w3389 -> [w3422 w3423]
              tunnel: [w3421 w3423] -> w3388
              frame False {
                n1398 = Create Folder(path (use dialog)=w3422) -> (created path=w3421:path)  [unwired: 2 in, 2 out]
              }
              frame True {
              }
            }
            n1399 = Number To Fractional String(number=w3397, precision (6)=i16 3) -> (F-format string=w3396:string)  [unwired: 2 in]
            n1400 = Format Date/Time String(seconds (now)=w3411, UTC format=TRUE) -> (date/time string=w3385:string)  [unwired: 1 in]
            "Start date" <- w3385
            n1401 = Format Date/Time String(seconds (now)=w3412, UTC format=TRUE) -> (date/time string=w3399:string)  [unwired: 1 in]
            "End date" <- w3399
            n1402 = Build Path(base path=w3388, name or relative path=w3386) -> (appended path=w3387:path)
            "File path" <- w3387
            n1403 = Format Into String(format string="%s %s;%s %s;%s %s;%s %s", "Start Date  ", w3385, "End Date", w3399, "Event Date", w3395, w3398, w3396) -> (resulting string=w3404:string)  [unwired: 2 in, 1 out]
            n1404 = Build Array(w3404) -> (w3405:string[])
            n1405 = call-poly <vilib>:"Write Delimited Spreadsheet.vi"("file path (dialog if empty)"=w3387, "1D data"=w3405, "append to file? (new file:F)"=TRUE, "transpose? (no:F)"=TRUE, "delimiter (\\t)"="\\t") -> ()  [unwired: 9 in, 2 out]
          }
          frame 6 {
            # "this block contain measure mode"
            # "loop to calculate timstamp (index)"
            # "this block contain measures+ time stamp which saved in the logfile"
            # "this block contain device type"
            # "this block contain time reference"
            # "logfile headers"
            n1406 = String Subset(string=w3443, offset (0)=0, length (rest)=16 ("length (rest)")) -> (substring=w3442:string)
            n1407 = call <vilib>:"Space Constant.vi"() -> ("String"=w3470:string)
            n1408 = String To Byte Array(string=w3577) -> (unsigned byte array=w3524:u8[])
            n1409 = Array Subset(array=w3524, index=10, length=4) -> (w3582:u8[])
            n1410 = Array To Cluster(array=w3524) -> (cluster=w3578:T15)
            n1411 = Array Subset(array=w3524, index=2, length=8) -> (w3585:u8[])
            n1412 = Array Subset(array=w3524, index=14, length=17) -> (w3523:u8[])
            n1413 = Array To Cluster(array=w3582) -> (cluster=w3581:T12)
            n1414 = Unbundle(w3578) -> ("unsigned byte array[0]"=w3500:u8, "unsigned byte array[1]"=w3520:u8)
            n1415 = Array To Cluster(array=w3585) -> (cluster=w3525:T12)
            n1416 = Array To Cluster(array=w3523) -> (cluster=w3574:T16)
            n1417 = Unbundle By Name(w3581) -> ("[0]"=w3580:u8)
            n1418 = Unbundle By Name(w3525) -> ("[0]"=w3530:u8, "[1]"=w3531:u8, "[2]"=w3534:u8, "[3]"=w3535:u8, "[4]"=w3528:u8, "[5]"=w3529:u8, "[6]"=w3537:u8, "[7]"=w3536:u8)
            n1419 = Unbundle By Name(w3574) -> ("[0]"=w3573:u8, "[1]"=w3572:u8, "[2]"=w3571:u8, "[3]"=w3568:u8, "[4]"=w3567:u8, "[5]"=w3565:u8, "[6]"=w3564:u8, "[7]"=w3563:u8, "[8]"=w3560:u8, "[9]"=w3559:u8, "[10]"=w3558:u8, "[11]"=w3555:u8, "[12]"=w3554:u8, "[13]"=w3550:u8, "[14]"=→"Network quality (LQI)":u8, "[15]"=→"channel that received alarm":u8)
            n1420 = Array Size(array=w3524) -> (size(s)=w3546:i32)
            n1421 = Join Numbers(hi=w3536, lo=w3537) -> ((hi.lo)=w3538:u16)
            n1422 = Join Numbers(hi=w3529, lo=w3528) -> ((hi.lo)=w3519:u16)
            "millisec" <- w3519
            n1423 = Join Numbers(hi=w3572, lo=w3573) -> ((hi.lo)=w3570:u16)
            n1424 = Join Numbers(hi=w3567, lo=w3568) -> ((hi.lo)=w3566:u16)
            n1425 = Join Numbers(hi=w3564, lo=w3565) -> ((hi.lo)=w3562:u16)
            n1426 = Join Numbers(hi=w3559, lo=w3560) -> ((hi.lo)=w3557:u16)
            n1427 = Join Numbers(hi=w3554, lo=w3555) -> ((hi.lo)=w3553:u16)
            n1428 = Equal To 0?(x=w3550) -> (x = 0?=→"not synchronised":bool)
            n1429 = Not Equal To 0?(x=w3550) -> (x != 0?=→"synchronised":bool)
            n1430 = To Word Integer(number=w3538) -> (16bit integer=w3440:i16)
            "Sampling rate" <- w3440
            n1431 = Subtract(x=w3546, y=30) -> (x-y=w3542:i32)
            n1432 = Join Numbers "date"(hi=w3535, lo=w3534) -> ((hi.lo)=w3533:u16)
            n1433 = Join Numbers "time"(hi=w3531, lo=w3530) -> ((hi.lo)=w3527:u16)
            n1434 = Divide(x=w3519, y=1000) -> (x/y=w3514:dbl)
            n1435 = Join Numbers(hi=w3571, lo=w3570) -> ((hi.lo)=w3569:u32)
            n1436 = Join Numbers(hi=w3563, lo=w3562) -> ((hi.lo)=w3561:u32)
            n1437 = Join Numbers(hi=w3558, lo=w3557) -> ((hi.lo)=w3556:u32)
            n1438 = To Unsigned Word Integer(number=w3514) -> (unsigned 16bit integer=w3518:u16)
            n1439 = To Unsigned Word Integer(number=w3533) -> (unsigned 16bit integer=w3494:u16)
            n1440 = To Word Integer(number=w3553) -> (16bit integer=→"Prev.number of daq per channel":i16)
            n1441 = To Word Integer(number=w3566) -> (16bit integer=w3521:i16)
            "Number of daq per channel" <- w3521
            n1442 = To Long Integer(number=w3556) -> (32bit integer=w3448:i32)
            "Data acquisition duration" <- w3448
            n1443 = To Long Integer(number=w3561) -> (32bit integer=w3449:i32)
            "Data notification cycle" <- w3449
            n1444 = Add(x=w3527, y=w3518) -> (x+y=w3495:u16)
            n1445 = Array Subset(array=w3524, index=30, length=w3542) -> (w3544:u8[])
            n1446 = To Long Integer(number=w3569) -> (32bit integer=w3522:i32)
            "Frame sequence Id" <- w3522
            n1447 = Join Numbers(hi=w3494, lo=w3495) -> ((hi.lo)=w3532:u32)
            n1448 = Decimate 1D Array(w3544) -> (w3539:u8[], w3543:u8[], w3541:u8[])
            n1449 = Number To Decimal String(number=w3449) -> (decimal integer string=w3458:string)  [unwired: 1 in]
            n1450 = Number To Decimal String(number=w3448) -> (decimal integer string=w3455:string)  [unwired: 1 in]
            n1451 = case shown="6" w3520 {
              tunnel: ["" "LDCDA mode" "Alarm mode" "Streaming mode" "Shock Detection mode" "LDC Math Result" "S_E_T" "Dynamic Math Result"] -> w3452
              frame Default {
              }
              frame 1 {
              }
              frame 2 {
              }
              frame 3 {
              }
              frame 4 {
              }
              frame 5 {
              }
              frame 6 {
              }
              frame 7 {
              }
            }
            "Measure mode" <- w3452
            n1452 = To Quad Integer(1:w3532) -> (0:w3515:i64)
            n1453 = Join Numbers(hi=w3543, lo=w3539) -> ((hi.lo)=w3540:u16[])
            n1454 = Multiply(x=w3521, y=w3522) -> (x*y=w3509:i32)
            n1455 = call "Unix Time to Timestamp.vi"("Fractional Second"=w3514, "Unix Time (s)"=w3515) -> ("Timestamp"=w3517:timestamp)  [unwired: 8 in, 1 out]
            n1456 = for {
              tunnel: w3541 -> [w3599] mode=indexing
              tunnel: [w3595] -> w3502 mode=indexing
              tunnel: w3540 -> [w3596] mode=indexing
              n1457 = To Word Integer(number=w3599) -> (16bit integer=w3597:i16)
              n1458 = Sign(1:w3597) -> (0:w3598:i16)
              n1459 = case shown="1" w3598 {
                tunnel: [_ w3601 w3604] -> w3595
                tunnel: w3596 -> [_ w3600 w3603]
                frame Default {
                }
                frame 1 {
                  n1460 = Divide(x=w3600, y=-1000.0) -> (x/y=w3601:dbl)
                }
                frame 0 {
                  n1461 = Divide(x=w3603, y=1000.0) -> (x/y=w3604:dbl)
                }
              }
            }
            n1462 = To Unsigned Quad Integer(1:w3509) -> (0:w3508:u64)
            n1463 = To Double Precision Float(number=w3440) -> (double precision float=w3492:dbl)
            n1464 = Increment(x=w3508) -> (x+1=w3510:u64)
            n1465 = Number To Decimal String(number=w3440) -> (decimal integer string=w3461:string)  [unwired: 1 in]
            n1466 = Format Date/Time String(time format string (%c)="%x %X %3u", seconds (now)=w3517, UTC format=TRUE) -> (date/time string=w3450:string)
            "Ref time" <- w3450
            n1467 = for {
              N: w3510 -> [_]
              tunnel: w3508 -> [w3594]
              tunnel: [w3594] -> w3512
            }
            n1468 = Decrement(x=w3512) -> (x-1=w3511:u64)
            n1469 = To Unsigned Byte Integer(number=w3580) -> (unsigned 8bit integer=w3439:u8)
            n1470 = case shown="5" w3500 {
              tunnel: ["AX-3D" "HI_INC_MONO" "HI_INC_BI" "X_INC_MONO " "X _INC_BI " "AX_3DS" ""] -> w3451
              frame 1 {
              }
              frame 2 {
              }
              frame 3 {
              }
              frame 4 {
              }
              frame 5 {
              }
              frame 6 {
              }
              frame Default {
              }
            }
            "Device type" <- w3451
            n1471 = Search and Replace String(replace all?=TRUE ("replace all? (F)"), input string=w3450, search string=":", replace string="_") -> (result string=w3479:string)  [unwired: 4 in, 3 out]
            n1472 = Search and Replace String(replace all?=TRUE ("replace all? (F)"), input string=w3479, search string=",", replace string="_") -> (result string=w3478:string)  [unwired: 4 in, 3 out]
            n1473 = Search and Replace String(replace all?=TRUE ("replace all? (F)"), input string=w3478, search string="/", replace string="_") -> (result string=w3474:string)  [unwired: 4 in, 3 out]
            n1474 = Concatenate Strings("Device type :", w3451, ";", "Measure Mode :", w3452, ";", "Time reference :" ("string"), w3450, ";", " Sampling rate :", w3461, ";" ("string"), "Data acquisition cycle :" ("string"), w3458, ";" ("string"), "Data acquisition duration :" ("string"), w3455, ";" ("string"), "\n") -> (w3468:string)
            n1475 = for {
              tunnel: w3502 -> [w3591] mode=indexing
              shift-right: [w3593] -> _
              shift-left: w3511 -> [w3590]
              tunnel: [w3592] -> w3493 mode=indexing
              tunnel: [w3591] -> _ mode=indexing
              n1476 = Increment(x=w3590) -> (x+1=w3593:u64)
              n1477 = To Unsigned Quad Integer(1:w3593) -> (0:w3592:u64)
            }
            n1478 = Build Array(w3468) -> (w3446:string[])
            n1479 = String Subset(string=w3474, offset (0)=0, length (rest)=20 ("length (rest)")) -> (substring=w3471:string)
            n1480 = Concatenate Strings(w3471, "_" ("string"), w3442, w3470) -> (w3447:string)
            n1481 = case shown="1" w3439 {
              tunnel: ["" "no active channel" "chZ " "chX " "chZ & chX " "chY" "chZ & chY" "chX & chY " "chZ& chX& chY " "INC_X" "chZ & INC_X " "chX & INC_X " "chZ& chX & INC_X " "chY & INC_X " "chZ  & chY & INC_X are activated " "chX  & chY & INC_X " "chZ& chX  & chY & INC_X " "INC_Y  " " chZ & INC_Y " " chX & INC_Y" "chZ & chX & INC_Y " " chY & INC_Y" "chZ & chY & INC_Y" "chX & chY & INC_Y " " chZ &chX & chY & INC_Y " " INC_X & INC_Y " "chZ &   INC_X & INC_Y " "chX & INC_X & INC_Y " " chZ & chX &  INC_X & INC_Y " " chY &  INC_X & INC_Y " "chZ & chY &  INC_X & INC_Y " "chX & chY &  INC_X & INC_Y " "chZ & chX & chY &  INC_X & INC_Y  "] -> w3579
              tunnel: w3502 -> [_ _ w3657 w3716 w3777 w3839 w3901 w3966 w4034 w4099 w4161 w4226 w4294 w4362 w4430 w4501 w4575 w4643 w4705 w4769 w4837 w4904 w4972 w5043 w5114 w5183 w5249 w5318 w5389 w5461 w5532 w5606 w5682]
              tunnel: [_ _ w3654 w3713 w3773 w3836 w3899 w3962 w4030 w4098 w4158 w4224 w4290 w4358 w4426 w4496 w4570 w4640 w4702 w4766 w4834 w4901 w4969 w5040 w5109 w5179 w5245 w5314 w5388 w5456 w5529 w5600 w5675] -> w3503
              tunnel: w3493 -> [_ _ w3656 w3715 w3776 w3837 w3900 w3965 w4029 w4097 w4159 w4225 w4293 w4361 w4429 w4500 w4574 w4642 w4704 w4768 w4836 w4903 w4971 w5041 w5110 w5182 w5248 w5315 w5385 w5460 w5531 w5604 w5677]
              tunnel: [_ _ w3653 _ w3772 _ w3896 _ w4028 _ w4156 _ w4288 _ w4424 _ w4568 _ w4700 _ w4831 _ w4966 _ w5107 _ w5243 _ w5382 _ w5525 _ w5674] -> w3501
              tunnel: [_ _ _ w3712 w3771 _ _ w3961 w4027 _ _ w4221 w4287 _ _ w4495 w4567 _ _ w4764 w4830 _ _ w5037 w5106 _ _ w5312 w5381 _ _ w5599 w5673] -> w3499
              tunnel: [_ _ _ _ _ w3835 w3895 w3960 w4026 _ _ _ _ w4357 w4423 w4494 w4566 _ _ _ _ w4899 w4965 w5036 w5105 _ _ _ _ w5455 w5524 w5598 w5672] -> w3498
              tunnel: [_ _ _ _ _ _ _ _ _ w4095 w4155 w4220 w4286 w4356 w4422 w4493 w4565 _ _ _ _ _ _ _ _ w5178 w5242 w5311 w5380 w5454 w5523 w5597 w5671] -> w3497
              tunnel: [_ _ _ _ _ _ _ _ _ _ _ _ _ _ _ _ _ w4639 w4699 w4763 w4829 w4898 w4964 w5035 w5104 w5177 w5241 w5310 w5379 w5453 w5522 w5596 w5670] -> w3496
              tunnel: w3495 -> [_ _ w3652 w3710 w3769 w3833 w3893 w3958 w4024 w4093 w4153 w4218 w4284 w4354 w4420 w4491 w4563 w4637 w4697 w4761 w4827 w4896 w4962 w5033 w5102 w5175 w5239 w5308 w5377 w5451 w5520 w5594 w5668]
              tunnel: w3494 -> [_ _ w3651 w3711 w3770 w3834 w3894 w3959 w4025 w4094 w4154 w4219 w4285 w4355 w4421 w4492 w4564 w4638 w4698 w4762 w4828 w4897 w4963 w5034 w5103 w5176 w5240 w5309 w5378 w5452 w5521 w5595 w5669]
              tunnel: w3493 -> [_ _ w3650 w3709 w3768 w3832 w3892 w3957 w4023 w4092 w4152 w4217 w4283 w4353 w4419 w4490 w4562 w4636 w4696 w4760 w4826 w4895 w4961 w5032 w5101 w5174 w5238 w5307 w5376 w5450 w5519 w5593 w5667]
              tunnel: w3492 -> [_ _ w3649 w3708 w3767 w3831 w3891 w3956 w4022 w4091 w4151 w4216 w4282 w4352 w4418 w4489 w4561 w4635 w4695 w4759 w4825 w4894 w4960 w5031 w5100 w5173 w5237 w5306 w5375 w5449 w5518 w5592 w5666]
              tunnel: [_ _ w3648 _ w3766 _ w3890 _ w4021 _ w4150 _ w4281 _ w4417 _ w4560 _ w4694 _ w4824 _ w4959 _ w5099 _ w5236 _ w5374 _ w5517 _ w5665] -> w3491
              tunnel: [_ _ _ w3707 w3766 _ _ w3955 w4020 _ _ w4215 w4280 _ _ w4488 w4559 _ _ w4758 w4823 _ _ w5030 w5099 _ _ w5305 w5374 _ _ w5591 w5665] -> w3441
              tunnel: [_ _ _ _ _ w3830 w3889 w3954 w4019 _ _ _ _ w4351 w4416 w4487 w4558 _ _ _ _ w4893 w4958 w5029 w5099 _ _ _ _ w5448 w5517 w5591 w5665] -> w3490
              tunnel: [_ _ _ _ _ _ _ _ _ w4090 w4149 w4214 w4279 w4350 w4415 w4486 w4557 _ _ _ _ _ _ _ _ w5172 w5236 w5305 w5374 w5448 w5517 w5591 w5665] -> w3489
              tunnel: [_ _ _ _ _ _ _ _ _ _ _ _ _ _ _ _ _ w4634 w4693 w4758 w4822 w4893 w4957 w5028 w5099 w5172 w5236 w5305 w5374 w5448 w5517 w5591 w5665] -> w3487
              tunnel: w3447 -> [_ _ w3634 w3684 w3743 w3807 w3865 w3931 w3996 w4067 w4126 w4191 w4256 w4327 w4392 w4463 w4534 w4611 w4670 w4734 w4799 w4869 w4934 w5005 w5075 w5149 w5213 w5282 w5351 w5425 w5494 w5568 w5642]
              tunnel: [_ _ w3624 w3683 w3742 w3806 w3866 w3929 w3995 w4066 w4125 w4190 w4255 w4326 w4391 w4462 w4533 w4610 w4669 w4735 w4798 w4870 w4933 w5004 w5076 w5148 w5212 w5281 w5350 w5424 w5493 w5567 w5641] -> w3488
              tunnel: w3446 -> [_ _ w3623 w3682 w3741 w3805 w3864 w3930 w3994 w4065 w4124 w4189 w4254 w4325 w4390 w4461 w4532 w4609 w4668 w4733 w4797 w4868 w4932 w5003 w5074 w5147 w5211 w5280 w5349 w5423 w5492 w5566 w5640]
              frame Default {
              }
              frame 0 {
              }
              frame 1 {
                w3629 = T14 2 items=["User Home"=0, "User Desktop"=1, "User Documents"=2, "User Application Data"=3, "User Preferences"=4, "User Temporary"=5, "Public Documents"=6, "Public Application Data"=7, "Public Preferences"=8, "Public Cache"=13, "System Core Libraries"=9, "System Installed Libraries"=10, "Application Files"=11, "Boot Volume Root"=12] ("system directory type")
                n1482 = call <vilib>:"Get System Directory.vi"("system directory type"=w3629) -> ("system directory"=w3640:path)  [unwired: 10 in]
                n1483 = Decimate 1D Array(w3657) -> (w3655:dbl[])
                n1484 = for {
                  tunnel: w3655 -> [w3676] mode=indexing
                  tunnel: [w3679] -> w3654 mode=indexing
                  tunnel: w3656 -> [w3678] mode=indexing
                  tunnel: [w3676] -> w3653 mode=indexing
                  tunnel: w3652 -> [w3671]
                  tunnel: w3651 -> [w3670]
                  tunnel: w3650 -> [w3669] mode=indexing
                  tunnel: w3649 -> [w3668]
                  tunnel: [w3663] -> w3648
                  n1485 = Join Numbers(hi=w3670, lo=w3671) -> ((hi.lo)=w3673:u32)
                  n1486 = Number To Fractional String(number=w3676, precision (6)=i16 3 ("width (-)")) -> (F-format string=w3680:string)  [unwired: 2 in]
                  n1487 = To Double Precision Float(number=w3669) -> (double precision float=w3674:dbl)
                  n1488 = To Unsigned Quad Integer(1:w3673) -> (0:w3672:u64)
                  n1489 = Divide(x=w3674, y=w3668) -> (x/y=w3675:dbl)
                  n1490 = call "Unix Time to Timestamp.vi"("Fractional Second"=w3675, "Unix Time (s)"=w3672) -> ("Timestamp"=w3662:timestamp)  [unwired: 8 in, 1 out]
                  n1491 = Number To Decimal String(number=w3678) -> (decimal integer string=w3677:string)  [unwired: 1 in]
